vi "probe_channels.vi"(8 "error in (no error)":errorcluster, 11 "TempProbeSet in":refnum<class "TempProbeSet.lvclass">) -> (0 "error out":errorcluster, 1 "number of channels":dbl, 2 "channels":string, 3 "TempProbeSet out":refnum<class "TempProbeSet.lvclass">)   [LabVIEW 2010, in "TempProbeSet.lvclass"]
uses:
  TempProbeSet.lvclass
  TempProbe.lvclass
  accessors/read_probes.vi
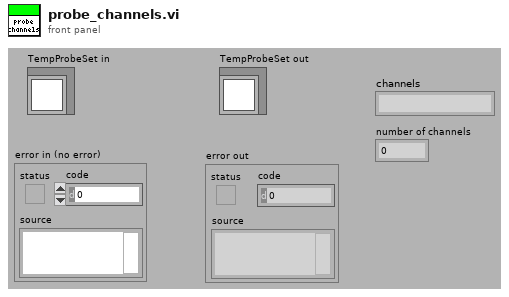
[diagram p1: front panel]
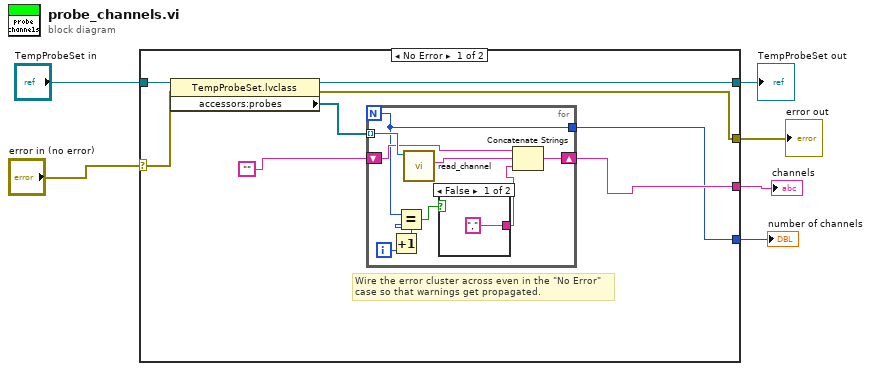
[diagram p0: block diagram]
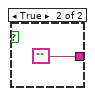
[diagram p2: hidden frame]
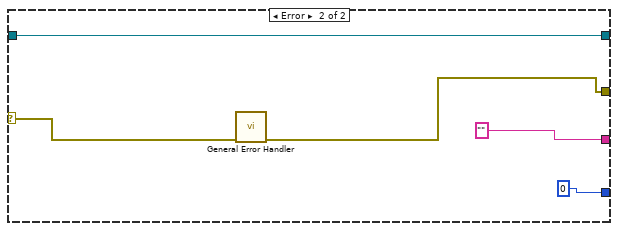
[diagram p3: hidden frame]
diagram:
  n1 = case shown="No Error" "error in (no error)" {
    selector: "error in (no error)" -> [w12 w28]
    tunnel: [w11 w30] -> w4
    tunnel: "TempProbeSet in" -> [w13 w30]
    tunnel: [w9 ""] -> w3
    tunnel: [w8 w27] -> w2
    tunnel: [w7 0] -> w1
    frame No Error {
      # "Wire the error cluster across even in the \"No Error\"\ncase so that warnings get propagated."
      n2 = property class="TempProbeSet.lvclass"(reference=w13, error in=w12) -> (reference out=w11:refnum<class "TempProbeSet.lvclass">, error out=w8:errorcluster, "accessors:probes"=w10:refnum<class "TempProbe.lvclass">[])
      n3 = for {
        N -> [w17]
        tunnel: w10 -> [w23] mode=indexing
        tunnel: [w17] -> w7
        shift-right: [w18] -> w9
        shift-left: "" -> [w19]
        i -> [w16]
        n4 = Increment(x=w16) -> (x+1=w15:i32)
        n5 = Equal?(x=w17, y=w15) -> (x = y?=w22:bool)
        n6 = call "read_channel.vi"("TempProbe in"=w23) -> ("Channel"=w21:string)  [unwired: 8 in, 2 out]
        n7 = case shown="False" w22 {
          tunnel: ["," ""] -> w20
          frame False {
          }
          frame True {
          }
        }
        n8 = Concatenate Strings(w19, w21, w20) -> (w18:string)
      }
    }
    frame Error {
      n9 = call <vilib>:"General Error Handler.vi"("error in (no error)"=w28) -> ("error out"=w27:errorcluster)  [unwired: 10 in, 4 out]
    }
  }
  "error out" <- w2
  "TempProbeSet out" <- w4
  "channels" <- w3
  "number of channels" <- w1
